vi "Integral_generator.vi"(8 "error in (no error)":errorcluster, 10 "sampling info":cluster{"Fs":dbl, "#s":dbl}, 11 "Signal Type":enum16{"sine", "polynom", "exponential"}(ring)) -> (0 "error out":errorcluster, 2 "Signal out":waveform(dbl), 3 "integral out":waveform(dbl))   [LabVIEW 2023]
uses:
  <vilib>/Analysis/1siggen.llb/Ramp Pattern by Samples.vi
  <vilib>/Analysis/polynomials.llb/Create Polynomial From Roots (DBL).vi
  <vilib>/Analysis/polynomials.llb/Indefinite Integral of Polynomial (DBL).vi
  <vilib>/Analysis/polynomials.llb/Scalar Polynomial Evaluation (DBL).vi
  <vilib>/measure/NI_MABase.lvlib
  <vilib>/Analysis/NI_AALPro.lvlib
  <vilib>/Analysis/NI_AALBase.lvlib
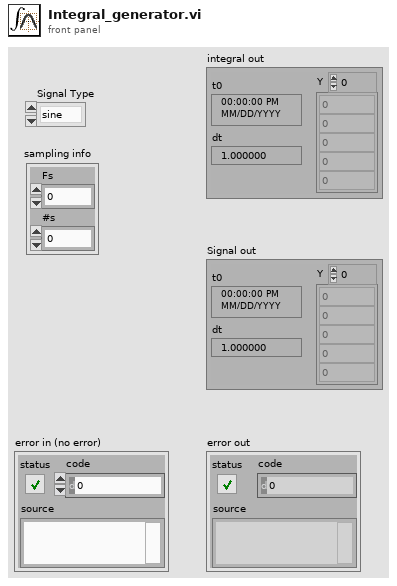
[diagram p1: front panel]
types:
  T1 = enum16{"Sine Wave", "Triangle Wave", "Square Wave", "Sawtooth Wave"}
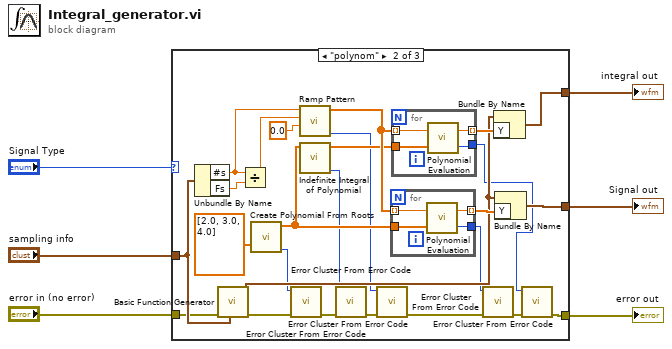
[diagram p0: block diagram]
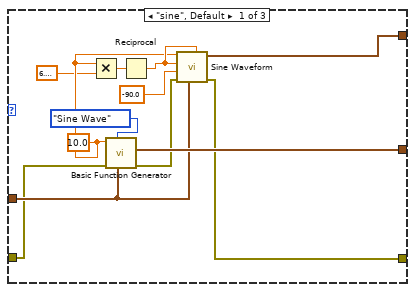
[diagram p2: hidden frame]
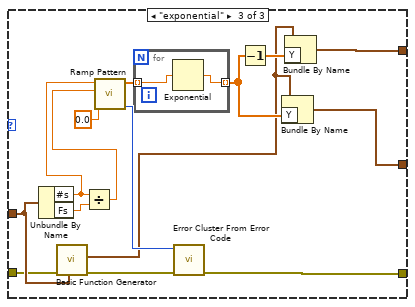
[diagram p3: hidden frame]
diagram:
  n1 = case shown="\"polynom\"" "Signal Type" {
    tunnel: "sampling info" -> [w10 w34 w59]
    tunnel: [w17 w37 w65] -> w2
    tunnel: [w13 w35 w62] -> w3
    tunnel: "error in (no error)" -> [w9 w30 w57]
    tunnel: [w7 w19 w54] -> w6
    frame "sine", Default {
      w12 = 10.0 ("frequency")
      n2 = Multiply(x=w12, y=6.283185307179586) -> (x*y=w15:dbl)
      n3 = call <vilib>:"Basic Function Generator.vi"("sampling info"=w10, "signal type"=T1."Sine Wave", "error in (no error)"=w9, "frequency"=w12) -> ("error out"=w8:errorcluster, "signal out"=w17:waveform(dbl))  [unwired: 5 in, 1 out]
      n4 = Reciprocal(x=w15) -> (1/x=w16:dbl)
      n5 = call <vilib>:"Sine Waveform.vi"("offset"=w16, "sampling info"=w10, "error in (no error)"=w8, "phase"=-90.0, "amplitude"=w16, "frequency"=w12) -> ("error out"=w7:errorcluster, "signal out"=w13:waveform(dbl))  [unwired: 4 in]
    }
    frame "polynom" {
      n6 = Unbundle By Name(w34) -> ("#s"=w31:dbl, "Fs"=w32:dbl)
      n7 = call <vilib>:"Basic Function Generator.vi"("sampling info"=w34, "error in (no error)"=w30) -> ("error out"=w29:errorcluster, "signal out"=w36:waveform(dbl))  [unwired: 7 in, 1 out]
      n8 = Divide(x=w31, y=w32) -> (x/y=w33:dbl)
      n9 = call-poly <vilib>:"Create Polynomial From Roots.vi"("Roots"=dbl[] [2.0, 3.0, 4.0]) -> ("error"=w28:i32, "P(x)"=w40:dbl[])  [unwired: 9 in]
      n10 = call <vilib>:"Error Cluster From Error Code.vi"("error in (no error)"=w29, "error code (0)"=w28) -> ("error out"=w27:errorcluster)  [unwired: 7 in]
      n11 = call-poly <vilib>:"Ramp Pattern.vi"("start"=0.0, "end"=w33, "samples"=w31) -> ("error"=w24:i32, "Ramp Pattern"=w42:dbl[])  [unwired: 7 in]
      n12 = call-poly <vilib>:"Indefinite Integral of Polynomial.vi"("P(x)"=w40) -> ("error"=w26:i32, "Indefinite Integral of P(x)"=w41:dbl[])  [unwired: 9 in]
      n13 = call <vilib>:"Error Cluster From Error Code.vi"("error in (no error)"=w27, "error code (0)"=w26) -> ("error out"=w25:errorcluster)  [unwired: 7 in]
      n14 = call <vilib>:"Error Cluster From Error Code.vi"("error in (no error)"=w25, "error code (0)"=w24) -> ("error out"=w22:errorcluster)  [unwired: 7 in]
      n15 = for {
        tunnel: w40 -> [w52]
        tunnel: w42 -> [w51] mode=indexing
        tunnel: [w50] -> w38 mode=indexing
        tunnel: [w49] -> w23
        n16 = call-poly <vilib>:"Polynomial Evaluation.vi"("P(x)"=w52, "a"=w51) -> ("error"=w49:i32, "P(a)"=w50:dbl)
      }
      n17 = for {
        tunnel: w41 -> [w48]
        tunnel: w42 -> [w47] mode=indexing
        tunnel: [w46] -> w39 mode=indexing
        tunnel: [w45] -> w20
        n18 = call-poly <vilib>:"Polynomial Evaluation.vi"("P(x)"=w48, "a"=w47) -> ("error"=w45:i32, "P(a)"=w46:dbl)
      }
      n19 = call <vilib>:"Error Cluster From Error Code.vi"("error in (no error)"=w22, "error code (0)"=w23) -> ("error out"=w21:errorcluster)  [unwired: 7 in]
      n20 = Bundle By Name(cluster=w36, "Y"=w39) -> (w35:waveform(dbl))
      n21 = Bundle By Name(cluster=w36, "Y"=w38) -> (w37:waveform(dbl))
      n22 = call <vilib>:"Error Cluster From Error Code.vi"("error in (no error)"=w21, "error code (0)"=w20) -> ("error out"=w19:errorcluster)  [unwired: 7 in]
    }
    frame "exponential" {
      n23 = Unbundle By Name(w59) -> ("#s"=w60:dbl, "Fs"=w61:dbl)
      n24 = call <vilib>:"Basic Function Generator.vi"("sampling info"=w59, "error in (no error)"=w57) -> ("error out"=w55:errorcluster, "signal out"=w53:waveform(dbl))  [unwired: 7 in, 1 out]
      n25 = Divide(x=w60, y=w61) -> (x/y=w58:dbl)
      n26 = call-poly <vilib>:"Ramp Pattern.vi"("start"=0.0, "end"=w58, "samples"=w60) -> ("error"=w56:i32, "Ramp Pattern"=w66:dbl[])  [unwired: 7 in]
      n27 = for {
        tunnel: w66 -> [w69] mode=indexing
        tunnel: [w68] -> w64 mode=indexing
        n28 = Exponential(1:w69) -> (0:w68:dbl)
      }
      n29 = call <vilib>:"Error Cluster From Error Code.vi"("error in (no error)"=w55, "error code (0)"=w56) -> ("error out"=w54:errorcluster)  [unwired: 7 in]
      n30 = Decrement(x=w64) -> (x-1=w63:dbl[])
      n31 = Bundle By Name(cluster=w53, "Y"=w64) -> (w65:waveform(dbl))
      n32 = Bundle By Name(cluster=w53, "Y"=w63) -> (w62:waveform(dbl))
    }
  }
  "error out" <- w6
  "integral out" <- w3
  "Signal out" <- w2
